vi "Tester.vi"() -> ()   [LabVIEW 2024, in "IPE Optimization Tester.lvlib"]
uses:
  IPE Optimization Tester.lvlib
  Tests/tests--enum.ctl
  <vilib>/Utility/High Resolution Relative Seconds.vi
  <vilib>/Analysis/baseanly.llb/Std Deviation and Variance.vi
  6a2990ba-c84e-4b58-bcba-cc98595d463d.vi
  592e4032-96de-47b5-8d28-165e25ce4dc9.vi
  42325635-cb82-47b4-8f32-23121f20b876.vi
  c979cdd8-d9da-4b6b-a4e0-95f4a3951907.vi
  c802cab8-e1c0-41dc-9a10-648cec1b264a.vi
  449d3225-5d58-48f7-9bf6-f925d79a1732.vi
  46b2c39e-2e50-4db4-89df-988747fec981.vi
  6048c143-94b8-4e20-9c50-857e2b8988b4.vi
panel:
  in  "Packet Size":i32=5000 caption="Numeric"
  in  "Copy Data":bool
  in  "Copy Results":bool
  out "Tests":T1[](array[typedef])
  out "Test Results":dbl[][](array[numeric]) format="%_4p"
  out "Raw Data":dbl[][](graph)
  out "Result":dbl[](array[numeric])
  in  "Data Size":i32=12000 caption="Numeric"
  in  "Test":T1
  in  "Reset":bool
  in  "Run":bool
  in  "Num of Calls":i32=1000 caption="Numeric"
  # "Mean (s)"
  # "StDev"
  # "Max (s)"
  # "Min (s)"
  # "Always wire up the final output to keep the compiler from being too smart thinking the data's never used so why bother"
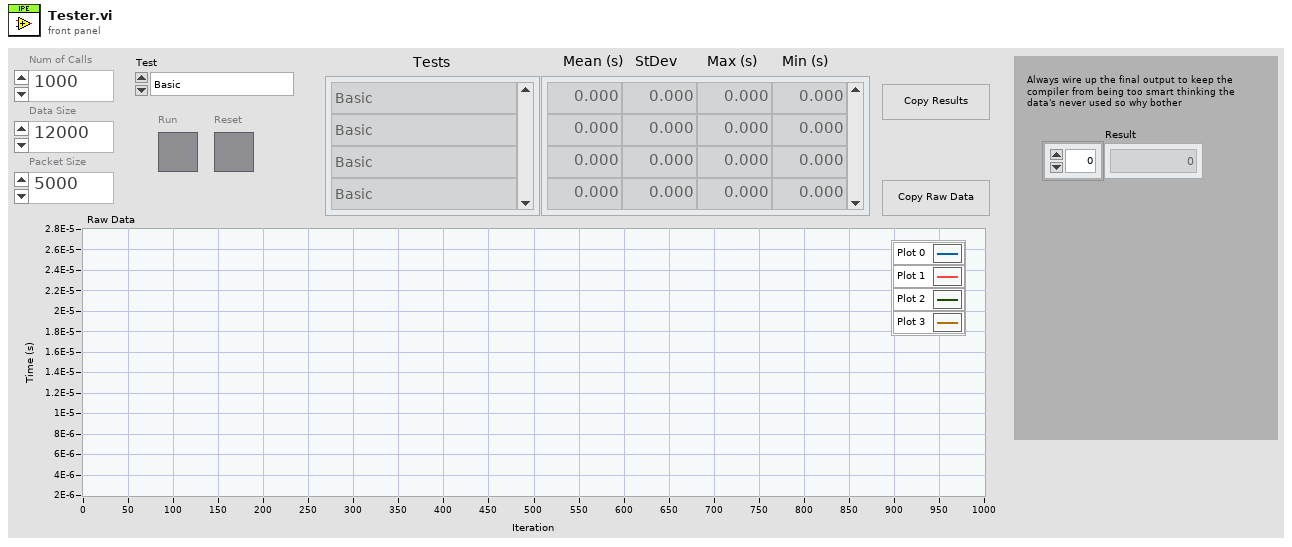
[diagram p1: front panel]
types:
  T1 = typedef "IPE Optimization Tester.lvlib/tests--enum.ctl" = enum16{"Basic", "Swap Inside", "Swap Outside", "Not Used yet"}
  T2 = typedef "IPE Optimization Tester.lvlib/data_bus--cluster.ctl" = cluster{"data":dbl[], "channels":string[]}
  T3 = typedef "IPE Optimization Tester.lvlib/test_data--cluster.ctl" = cluster{"data":dbl[], "encoded packets":string[], "packet size":i32}
  T4 = typedef "test_data--cluster.ctl" = cluster{"Tests":T1[], "results":dbl[][], "raw_data":dbl[][]}
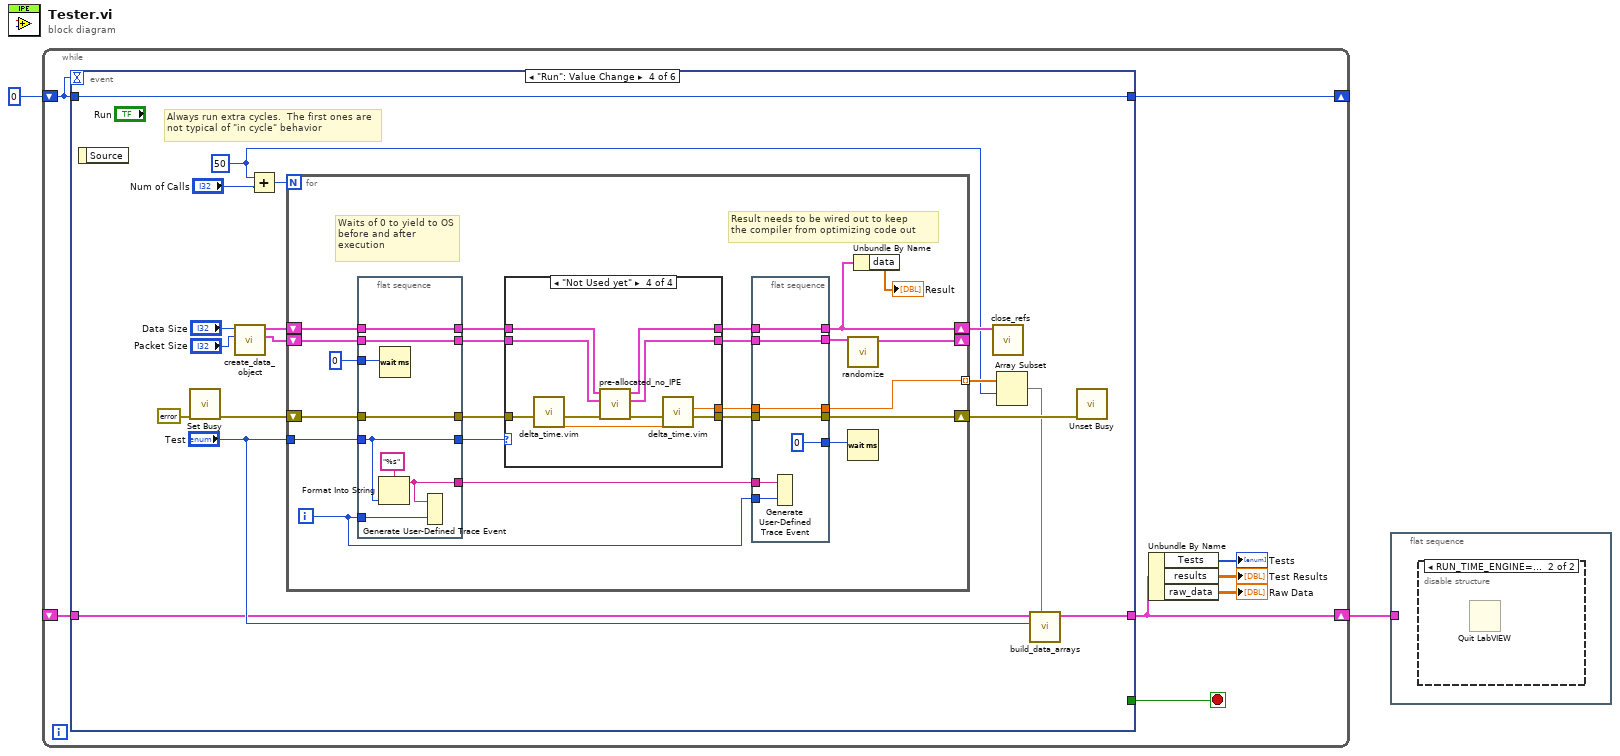
[diagram p0: block diagram]
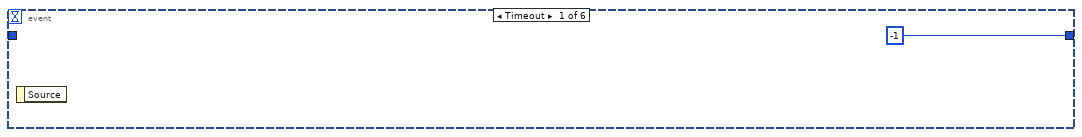
[diagram p3: hidden frame]
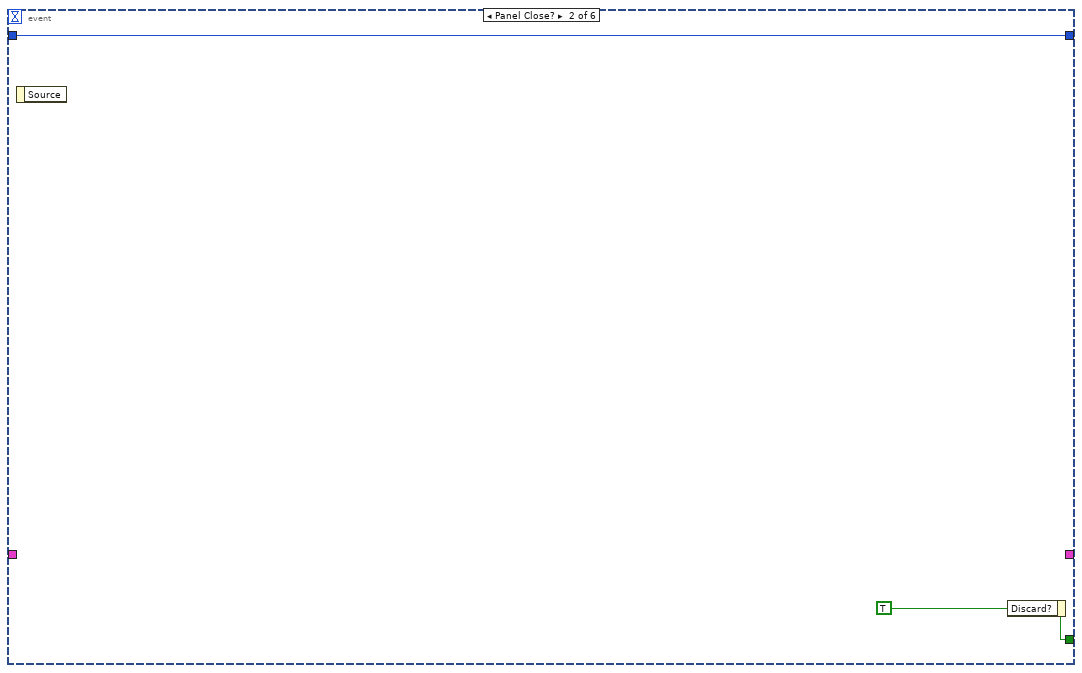
[diagram p4: hidden frame]
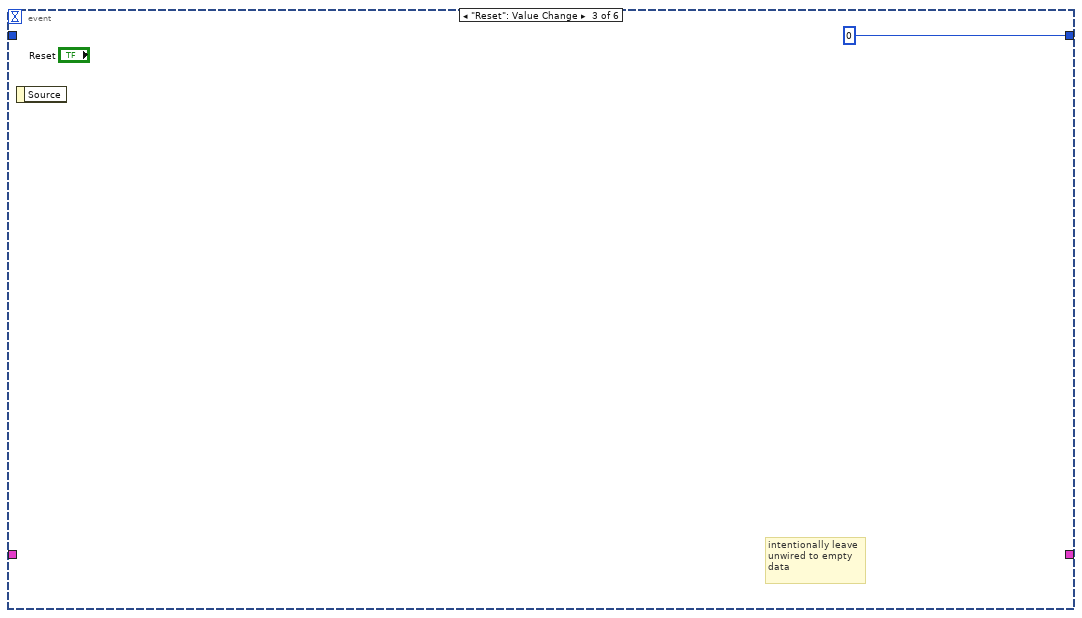
[diagram p5: hidden frame]
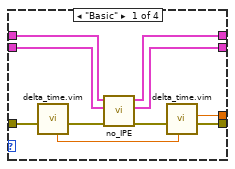
[diagram p6: hidden frame]
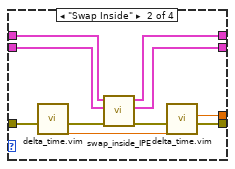
[diagram p7: hidden frame]
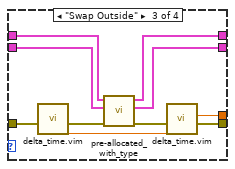
[diagram p8: hidden frame]
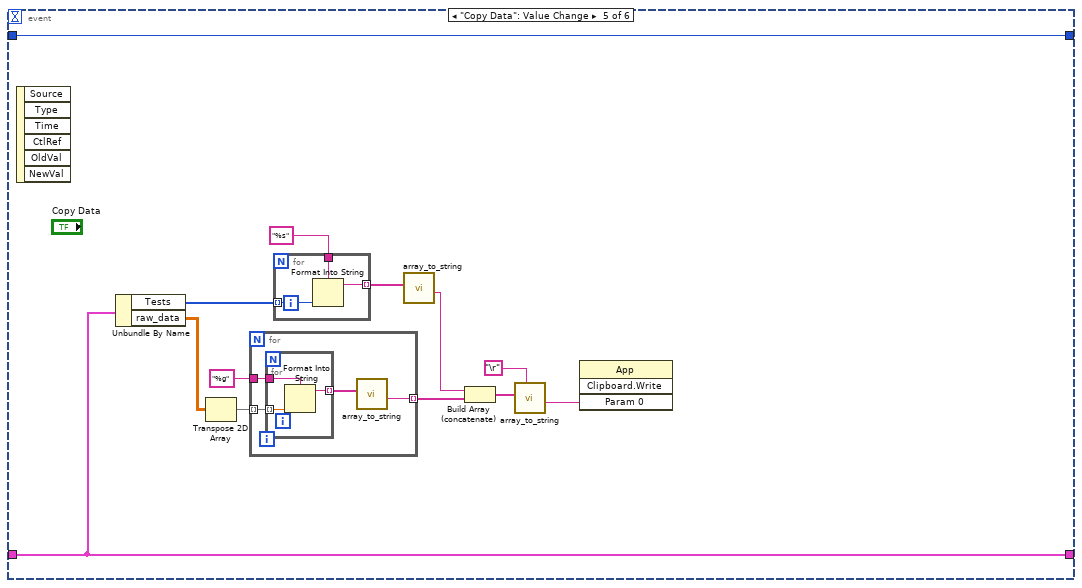
[diagram p9: hidden frame]
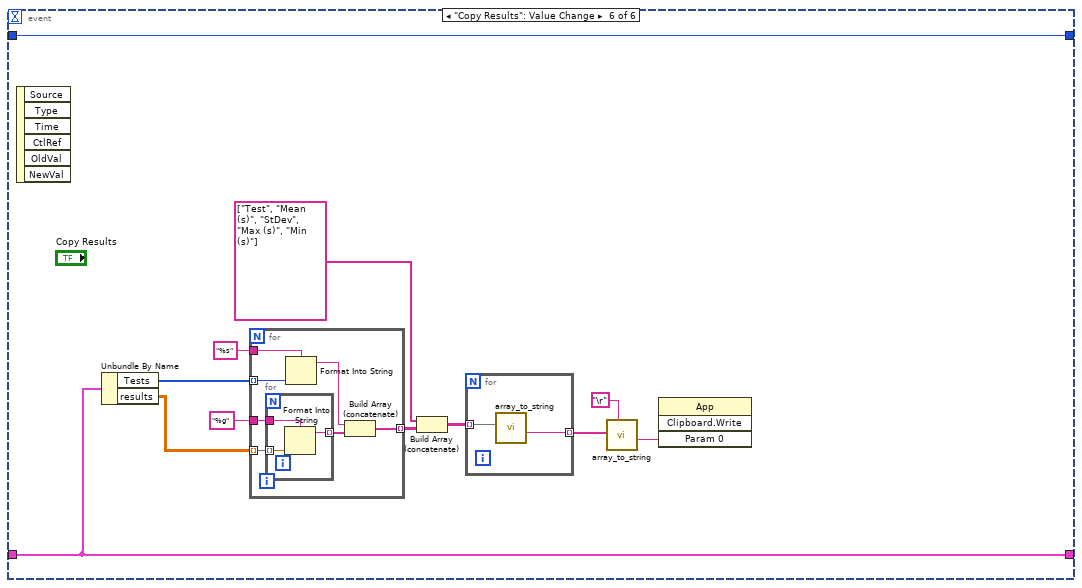
[diagram p10: hidden frame]
diagram:
  n1 = while {
    shift-right: [w9] -> _
    shift-left: 0 -> [w10]
    shift-right: [w6] -> w1
    shift-left: _ -> [w7]
    stop <- w8 stop-if-true
    n2 = event shown="[3] \"Run\": Value Change" {
      selector: _ -> [_ _ _ _ _ _]
      dyn-events: _ -> [_ _ _ _ _ _]
      timeout: w10 -> [_ _ _ _ _ _]
      tunnel: w10 -> [_ w13 _ w31 w121 w143]
      tunnel: [-1 w13 0 w31 w121 w143] -> w9
      tunnel: [_ w12 _ _ _ _] -> w8
      tunnel: w7 -> [_ _ _ w16 w111 w134]
      tunnel: [_ _ _ w17 w111 w134] -> w6
      event Timeout {
        n3 = event-data() -> ()  [unwired: 1 in, 1 out]
      }
      event Panel Close? {
        w12 = TRUE ("Discard?")
        n4 = event-data() -> ()  [unwired: 1 in, 1 out]
        n5 = event-data("Discard?"=w12) -> ()  [unwired: 1 in, 1 out]
      }
      event "Reset": Value Change {
        # "intentionally leave\nunwired to empty\ndata"
        n6 = event-data() -> ()  [unwired: 1 in, 1 out]
      }
      event "Run": Value Change {
        w22 = 50 ("x")
        # "Always run extra cycles.  The first ones are not typical of \"in cycle\" behavior"
        n7 = event-data() -> ()  [unwired: 1 in, 1 out]
        n8 = call <vilib>:"Set Busy.vi"("error in (no error)"=errorcluster {"status"=FALSE, "code"=0, "source"=""}) -> ("error out"=w28:errorcluster)  [unwired: 9 in, 1 out]
        n9 = call "create_data_object.vi"("Packet Size"="Packet Size", "data size"="Data Size") -> ("data bus"=w15:T2, "Test Data"=w29:T3)  [unwired: 8 in]
        n10 = Add(x=w22, y="Num of Calls") -> (x+y=w23:i32)
        n11 = for {
          N: w23 -> [_]
          shift-right: [w33] -> w25
          shift-left: w29 -> [w51]
          shift-right: [w48] -> w27
          shift-left: w28 -> [w52]
          tunnel: "Test" -> [w53]
          tunnel: [w45] -> w26 mode=indexing
          shift-right: [w34] -> _
          shift-left: w15 -> [w38]
          i -> [w47]
          # "Waits of 0 to yield to OS before and after execution"
          # "Result needs to be wired out to keep\nthe compiler from optimizing code out"
          n12 = flat-sequence {
            tunnel: [w105] -> w46
            tunnel: w53 -> [w105]
            tunnel: w47 -> [w106]
            tunnel: [w108] -> w50
            tunnel: w52 -> [w108]
            tunnel: w51 -> [w107]
            tunnel: [w107] -> w43
            tunnel: [w103] -> w41
            tunnel: u32 0 -> [w102]
            tunnel: w38 -> [w101]
            tunnel: [w101] -> w37
            frame #0 {
              n13 = Format Into String(format string="%s", w105) -> (resulting string=w103:string)  [unwired: 2 in, 1 out]
              n14 = Wait (ms)(milliseconds to wait=w102) -> ()  [unwired: 1 out]
              n15 = Generate User-Defined Trace Event(1:w106, 2:w103) -> ()
            }
          }
          n16 = case shown="\"Not Used yet\"" w46 {
            tunnel: w50 -> [w66 w76 w86 w96]
            tunnel: [w63 w73 w83 w93] -> w49
            tunnel: [w69 w79 w89 w99] -> w44
            tunnel: w43 -> [w68 w78 w88 w98]
            tunnel: [w67 w77 w87 w97] -> w42
            tunnel: w37 -> [w62 w72 w82 w92]
            tunnel: [w61 w71 w81 w91] -> w36
            frame "Basic" {
              n17 = call "delta_time.vim"("inlined Input"=w66) -> ("inlined output"=w64:errorcluster, "Time out"=w70:dbl)  [unwired: 8 in, 1 out]
              n18 = call "no_IPE.vi"("error in (no error)"=w64, "data bus in"=w62, "Test Data in"=w68) -> ("error out"=w65:errorcluster, "data bus out"=w61:T2, "Test Data out"=w67:T3)  [unwired: 6 in]
              n19 = call "delta_time.vim"("Time in"=w70, "inlined Input"=w65) -> ("inlined output"=w63:errorcluster, "Delta Time"=w69:dbl)  [unwired: 7 in, 1 out]
            }
            frame "Swap Inside" {
              n20 = call "delta_time.vim"("inlined Input"=w76) -> ("inlined output"=w75:errorcluster, "Time out"=w80:dbl)  [unwired: 8 in, 1 out]
              n21 = call "swap_inside_IPE.vi"("error in (no error)"=w75, "data bus in"=w72, "Test Data in"=w78) -> ("error out"=w74:errorcluster, "data bus out"=w71:T2, "Test Data out"=w77:T3)  [unwired: 6 in]
              n22 = call "delta_time.vim"("Time in"=w80, "inlined Input"=w74) -> ("inlined output"=w73:errorcluster, "Delta Time"=w79:dbl)  [unwired: 7 in, 1 out]
            }
            frame "Swap Outside" {
              n23 = call "delta_time.vim"("inlined Input"=w86) -> ("inlined output"=w85:errorcluster, "Time out"=w90:dbl)  [unwired: 8 in, 1 out]
              n24 = call "pre-allocated_with_type.vi"("error in (no error)"=w85, "data bus in"=w82, "Test Data in"=w88) -> ("error out"=w84:errorcluster, "data bus out"=w81:T2, "Test Data out"=w87:T3)  [unwired: 6 in]
              n25 = call "delta_time.vim"("Time in"=w90, "inlined Input"=w84) -> ("inlined output"=w83:errorcluster, "Delta Time"=w89:dbl)  [unwired: 7 in, 1 out]
            }
            frame "Not Used yet" {
              n26 = call "delta_time.vim"("inlined Input"=w96) -> ("inlined output"=w95:errorcluster, "Time out"=w100:dbl)  [unwired: 8 in, 1 out]
              n27 = call "pre-allocated_no_IPE.vi"("error in (no error)"=w95, "data bus in"=w92, "Test Data in"=w98) -> ("error out"=w94:errorcluster, "data bus out"=w91:T2, "Test Data out"=w97:T3)  [unwired: 6 in]
              n28 = call "delta_time.vim"("Time in"=w100, "inlined Input"=w94) -> ("inlined output"=w93:errorcluster, "Delta Time"=w99:dbl)  [unwired: 7 in, 1 out]
            }
          }
          n29 = flat-sequence {
            tunnel: w47 -> [w60]
            tunnel: [w59] -> w48
            tunnel: w49 -> [w59]
            tunnel: w42 -> [w58]
            tunnel: [w58] -> w33
            tunnel: [w57] -> w45
            tunnel: w44 -> [w57]
            tunnel: w41 -> [w56]
            tunnel: [u32 0] -> w40
            tunnel: w36 -> [w54]
            tunnel: [w54] -> w35
            frame #0 {
              n30 = Generate User-Defined Trace Event(1:w60, 2:w56) -> ()
            }
          }
          n31 = call "randomize.vi"("data bus"=w35) -> ("data bus out"=w34:T2)  [unwired: 10 in]
          n32 = Wait (ms)(milliseconds to wait=w40) -> ()  [unwired: 1 out]
          n33 = Unbundle By Name(w33) -> ("data"=→"Result":dbl[])
        }
        n34 = call "close_refs.vi"("Test Data in"=w25) -> ()  [unwired: 11 in]
        n35 = Array Subset(array=w26, index=w22) -> (w19:dbl[])  [unwired: 1 in]
        n36 = call "build_data_arrays.vi"("last_test"=w19, "Test"="Test", "test_data in"=w16) -> ("test_data out"=w17:T4)  [unwired: 8 in]
        n37 = call <vilib>:"Unset Busy.vi"("error in (no error)"=w27) -> ()  [unwired: 10 in, 1 out]
      }
      event "Copy Data": Value Change {
        n38 = event-data() -> ()  [unwired: 1 in, 6 out]
        n39 = Unbundle By Name(w111) -> ("Tests"=w109:T1[], "raw_data"=w110:dbl[][])
        n40 = Transpose 2D Array(2D array=w110) -> (transposed array=w115:dbl[][])
        n41 = for {
          tunnel: w115 -> [w123] mode=indexing
          tunnel: [w125] -> w119 mode=indexing
          tunnel: "%g" -> [w122]
          n42 = for {
            tunnel: [w128] -> w124 mode=indexing
            tunnel: w123 -> [w126] mode=indexing
            tunnel: w122 -> [w127]
            n43 = Format Into String(format string=w127, w126) -> (resulting string=w128:string)  [unwired: 2 in, 1 out]
          }
          n44 = call "array_to_string.vi"("Array of Strings"=w124) -> ("delimited string"=w125:string)  [unwired: 10 in]
        }
        n45 = for {
          tunnel: "%s" -> [w131]
          tunnel: [w130] -> w113 mode=indexing
          tunnel: w109 -> [w129] mode=indexing
          n46 = Format Into String(format string=w131, w129) -> (resulting string=w130:string)  [unwired: 2 in, 1 out]
        }
        n47 = call "array_to_string.vi"("Array of Strings"=w113) -> ("delimited string"=w112:string)  [unwired: 10 in]
        n48 = Build Array (concatenate)(w112, w119) -> (w118:string[])
        n49 = call "array_to_string.vi"("delimiter (Tab)"="\r", "Array of Strings"=w118) -> ("delimited string"=w116:string)  [unwired: 9 in]
        n50 = invoke class="App" method="Clipboard.Write"("Param 0"=w116) -> ()  [unwired: 3 in, 4 out]
      }
      event "Copy Results": Value Change {
        n51 = event-data() -> ()  [unwired: 1 in, 6 out]
        n52 = Unbundle By Name(w134) -> ("Tests"=w133:T1[], "results"=w132:dbl[][])
        n53 = for {
          tunnel: [w148] -> w142 mode=indexing
          tunnel: "%g" -> [w152]
          tunnel: "%s" -> [w151]
          tunnel: w133 -> [w147] mode=indexing
          tunnel: w132 -> [w146] mode=indexing
          n54 = for {
            tunnel: [w155] -> w150 mode=indexing
            tunnel: w152 -> [w154]
            tunnel: w146 -> [w153] mode=indexing
            n55 = Format Into String(format string=w154, w153) -> (resulting string=w155:string)  [unwired: 2 in, 1 out]
          }
          n56 = Format Into String(format string=w151, w147) -> (resulting string=w149:string)  [unwired: 2 in, 1 out]
          n57 = Build Array (concatenate)(w149, w150) -> (w148:string[])
        }
        n58 = Build Array (concatenate)(string[] ["Test", "Mean (s)", "StDev", "Max (s)", "Min (s)"], w142) -> (w136:string[][])
        n59 = for {
          tunnel: w136 -> [w145] mode=indexing
          tunnel: [w144] -> w135 mode=indexing
          n60 = call "array_to_string.vi"("Array of Strings"=w145) -> ("delimited string"=w144:string)  [unwired: 10 in]
        }
        n61 = call "array_to_string.vi"("delimiter (Tab)"="\r", "Array of Strings"=w135) -> ("delimited string"=w140:string)  [unwired: 9 in]
        n62 = invoke class="App" method="Clipboard.Write"("Param 0"=w140) -> ()  [unwired: 3 in, 4 out]
      }
    }
    n63 = Unbundle By Name(w6) -> ("Tests"=→"Tests":T1[], "results"=→"Test Results":dbl[][], "raw_data"=→"Raw Data":dbl[][])
  }
  n64 = flat-sequence {
    tunnel: w1 -> [_]
    frame #0 {
      n65 = disable-structure shown="RUN_TIME_ENGINE==True" {
        frame condition #0 (active) {
        }
        frame condition #1 {
          n66 = Quit LabVIEW() -> ()  [unwired: 1 in]
        }
      }
    }
  }
